vi "(SubVI) WriteRead Waveform_YCC.vi"(4 "ADC Rate for 20bit (ms)":T1(ring)=enum."3750 Hz", 5 "Number of Positions to Read":u32=2 min=2 max=10000, 6 "Data Array In for writing":dbl[](array[numeric]) format="%.2f", 7 "DAC Rate (Write) (ms)":dbl=1.0 min=0.0333333 max=5.0 format="%.4f", 8 "Axis":u32, 9 "handle":i32) -> (1 "Data Array Out for reading":dbl[](array[numeric]) format="%.2f", 2 "Time array for reading":dbl[](array[numeric]))   [LabVIEW 2014]
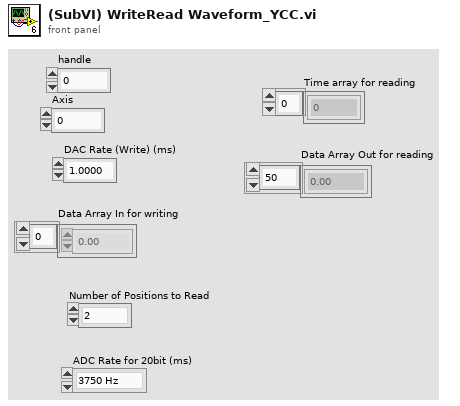
[diagram p1: front panel]
types:
  T1 = enum16{"50 Hz", "60 Hz", "100 Hz", "500 Hz", "1000 Hz", "2000 Hz", "3750 Hz"}
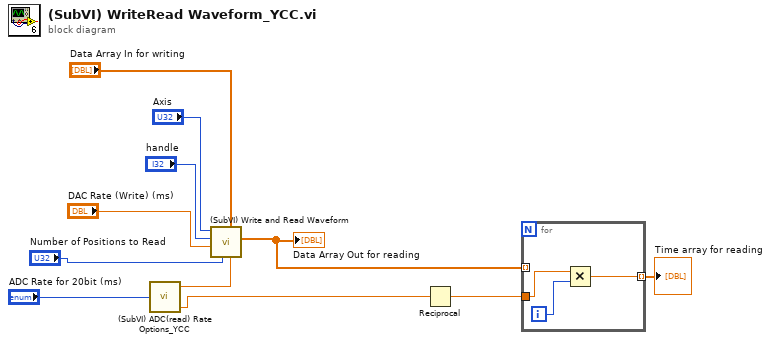
[diagram p0: block diagram]
diagram:
  n1 = call "(SubVI) ADC(read) Rate Options_YCC.vi"("ADC Rate for 20bit (ms)"="ADC Rate for 20bit (ms)") -> ("Sampling Rate for reading (Hz)"=w3:dbl, "waiting code for Reading (20bits)"=w11:dbl)  [unwired: 3 in]
  n2 = call "(SubVI) Write and Read Waveform.vi"("ADC Rate (Read)(ms)"=w11, "Data Array In to write"="Data Array In for writing", "Number of Positions to Read"="Number of Positions to Read", "DAC Rate (Write) (ms)"="DAC Rate (Write) (ms)", "handle"="handle", "Axis"="Axis") -> ("Data Array Out to read"=w4:dbl[])  [unwired: 5 in]
  "Data Array Out for reading" <- w4
  n3 = Reciprocal(x=w3) -> (1/x=w2:dbl)
  n4 = for {
    tunnel: w4 -> [_] mode=indexing
    tunnel: w2 -> [w13]
    tunnel: [w12] -> w1 mode=indexing
    i -> [w14]
    n5 = Multiply(x=w13, y=w14) -> (x*y=w12:dbl)
  }
  "Time array for reading" <- w1
